vi "SubTemplate2UI.vi"() -> ()   [LabVIEW 2016]
uses:
  Package ResourceControl/ViHandler/ViHandler.ViInfo.ctl
  Message Queue/private/MessageQueue.MessageTypeDef.ctl
  Package ErrorHandling/ErrorHandling.lvclass/ErrorHandling.ctl
  Package ErrorHandling/ErrorHandling.checkForErrorAndHandle.vi
  Package ErrorHandling/ErrorHandling.GetErrorHandler.vi
  <vilib>/Utility/error.llb/Clear Errors.vi
  StringFunctions/StringFunctions_ReplaceAllBlindSigns.vi
  <vilib>/dlg_ctls.llb/Space Constant.vi
  <vilib>/Utility/error.llb/Error Cluster From Error Code.vi
  TimingFunctions/TimingFunctions_getUtcTimestamp.vi
  <vilib>/Utility/error.llb/Trim Whitespace.vi
  <vilib>/Utility/error.llb/Search and Replace Pattern.vi
  Package ErrorHandling/ErrorHandling.addLastErrorToFile.vi
  <vilib>/ErrorRing/Error Ring.xnode
  Package ErrorHandling/ErrorHandling.lvclass
  Package ResourceControl/ViHandler/ViHandler.lvclass
panel:
  out "ViInfoTemp":T1
  # "Batch Conversion"
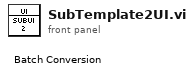
[diagram p1: front panel]
types:
  T1 = typedef "ViHandler.lvclass/ViHandler.ViInfo.ctl" = cluster{"ViName":string, "ViReference":refnum<vi>, "ViQueueName":string}
  T2 = typedef "MessageQueue.MessageTypeDef.ctl" = cluster{"Message":string, "Data":variant}
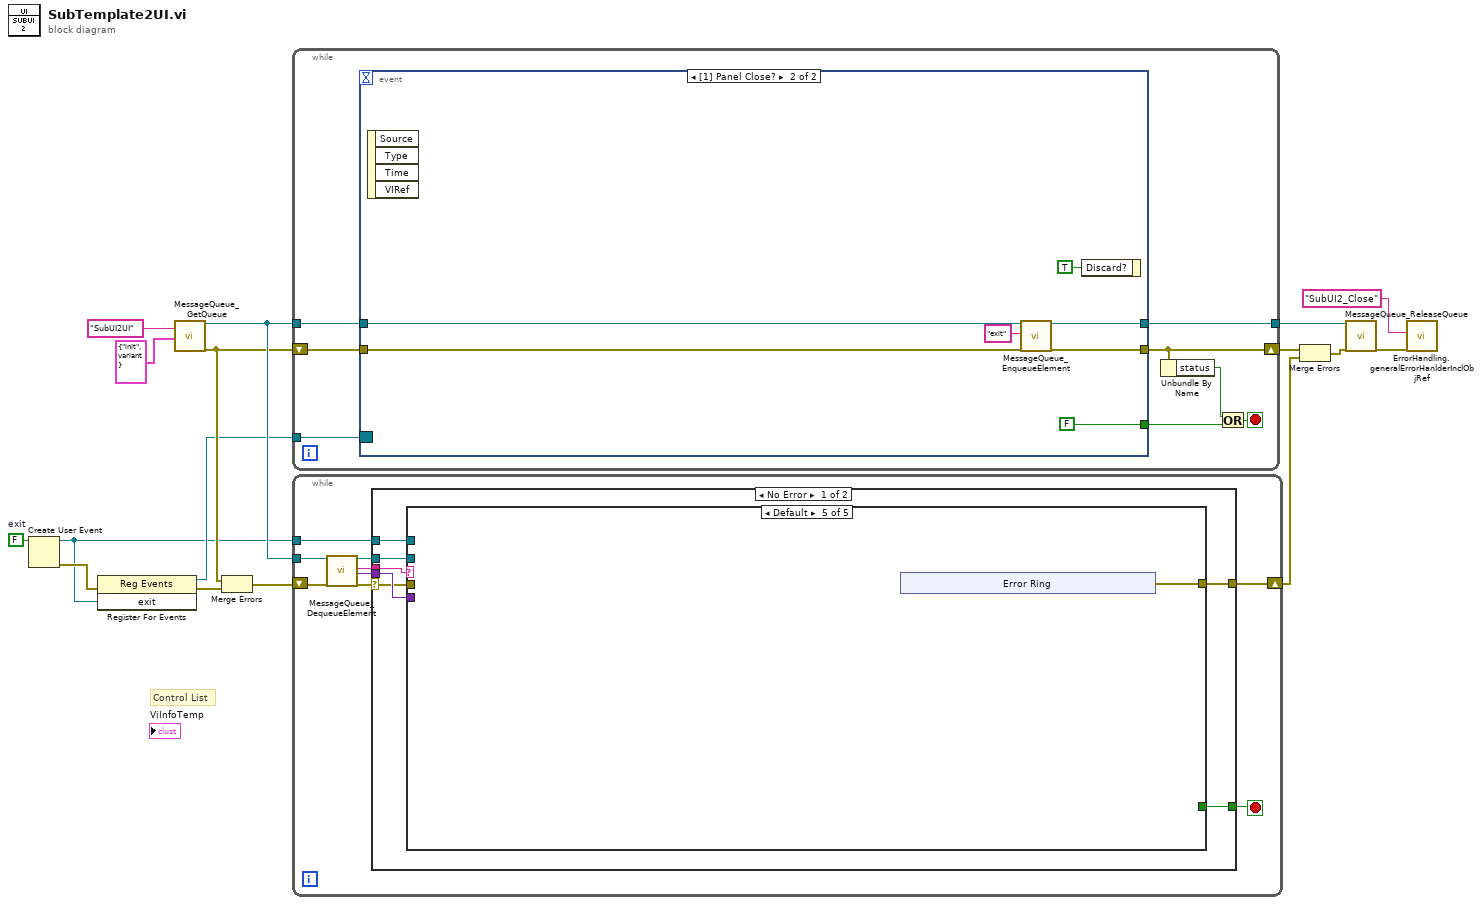
[diagram p0: block diagram]
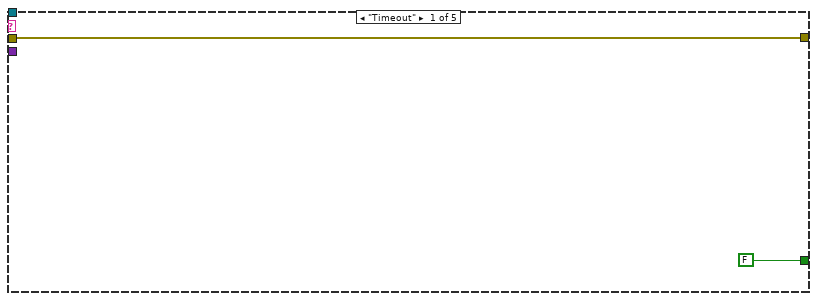
[diagram p2: hidden frame]
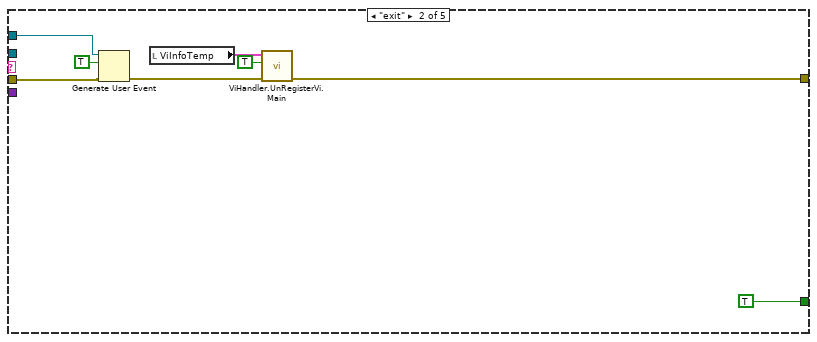
[diagram p3: hidden frame]
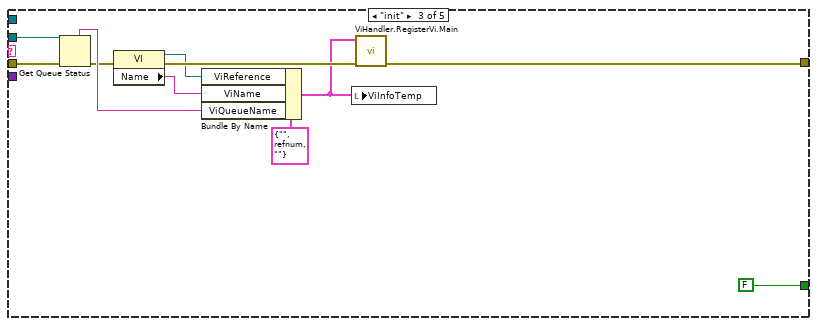
[diagram p4: hidden frame]
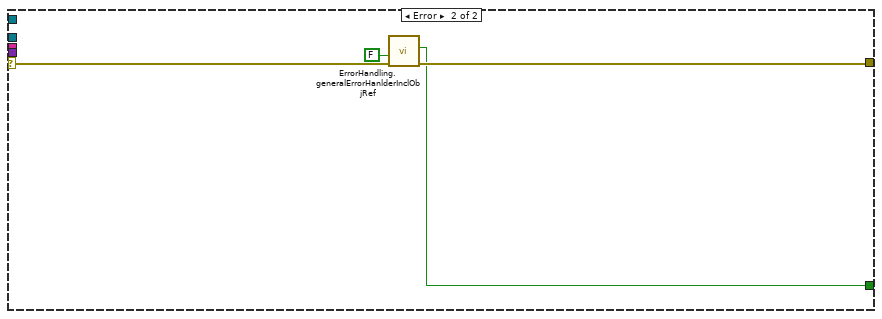
[diagram p6: hidden frame]
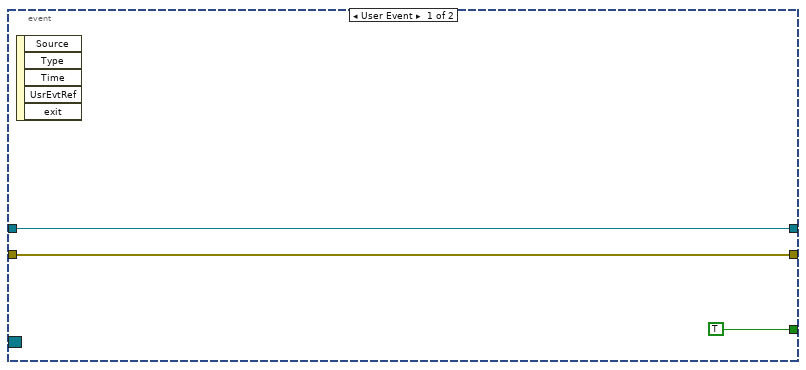
[diagram p7: hidden frame]
diagram:
  w9 = FALSE  # exit
  # "Control List"
  n1 = Create User Event(user event datatype=w9) -> (user event=w7:refnum<user-event>, error out=w8:errorcluster)  [unwired: 1 in]
  n2 = register-events(error in=w8, w7) -> (reference out=w11:refnum<event-registration>, error out=w13:errorcluster)  [unwired: 1 in]
  n3 = call "MessageQueue_GetQueue.vi"("Name"="SubUI2UI", "OptionalInitValue"=T2 {"Message"="init", "Data"=variant}) -> ("QueueOut"=w15:refnum<queue>, "ErrorOut"=w12:errorcluster)  [unwired: 15 in, 1 out]
  n4 = Merge Errors(w12, w13) -> (w10:errorcluster)
  n5 = while {
    tunnel: w15 -> [w24]
    tunnel: [w23] -> w16
    shift-right: [w20] -> w4
    shift-left: w12 -> [w22]
    tunnel: w11 -> [w17]
    stop <- w19 stop-if-true
    n6 = event shown="[1] Panel Close?" {
      selector: w17 -> [_ _]
      dyn-events: _ -> [_ _]
      timeout: _ -> [_ _]
      tunnel: w24 -> [w26 w34]
      tunnel: [w26 w33] -> w23
      tunnel: [w25 w32] -> w20
      tunnel: w22 -> [w25 w31]
      tunnel: [TRUE FALSE] -> w21
      event User Event {
        n7 = event-data() -> ()  [unwired: 1 in, 5 out]
      }
      event Panel Close? {
        n8 = event-data() -> ()  [unwired: 1 in, 4 out]
        n9 = call "MessageQueue_EnqueueElement.vi"("QueueIn"=w34, "Message"="exit", "ErrorIn"=w31) -> ("QueueOut"=w33:refnum<queue>, "ErrorOut"=w32:errorcluster)  [unwired: 15 in]
        n10 = event-data("Discard?"=TRUE) -> ()  [unwired: 1 in, 1 out]
      }
    }
    n11 = Unbundle By Name(w20) -> ("status"=w18:bool)
    n12 = Or(x=w18, y=w21) -> (x .or. y?=w19:bool)
  }
  n13 = while {
    tunnel: w15 -> [w43]
    tunnel: w7 -> [w36]
    shift-right: [w35] -> w5
    shift-left: w10 -> [w37]
    stop <- w38 stop-if-true
    n14 = call "MessageQueue_DequeueElement.vi"("QueueIn"=w43, "ErrorIn"=w37) -> ("QueueOut"=w41:refnum<queue>, "Message"=w40:string, "Data"=w39:variant, "ErrorOut"=w42:errorcluster)  [unwired: 13 in, 1 out]
    n15 = case shown="No Error" w42 {
      selector: w42 -> [w46 w82]
      tunnel: w41 -> [w50 _]
      tunnel: w40 -> [w49 _]
      tunnel: w39 -> [w48 _]
      tunnel: [w47 w80] -> w38
      tunnel: w36 -> [w45 _]
      tunnel: [w44 w81] -> w35
      frame No Error {
        n16 = case shown="Default" w49 {
          tunnel: w50 -> [_ _ w63 _ _]
          tunnel: w48 -> [_ _ _ _ _]
          tunnel: [FALSE TRUE FALSE _ _] -> w47
          tunnel: w46 -> [w51 w58 w64 w72 _]
          tunnel: w45 -> [_ w57 _ _ _]
          tunnel: [w51 w54 w61 w72 w73] -> w44
          frame "Timeout" {
          }
          frame "exit" {
            n17 = Generate User Event(user event=w57, event data cluster=TRUE ("event data"), error in=w58) -> (error out=w55:errorcluster)  [unwired: 1 in, 1 out]
            n18 = local read "ViInfoTemp"() -> (w56:T1)
            n19 = call "ViHandler.UnRegisterVi.Main.vi"("ErrorIn"=w55, "FinalExit?"=TRUE, "ViInfo"=w56) -> ("ErrorOut"=w54:errorcluster)  [unwired: 7 in, 1 out]
          }
          frame "init" {
            n20 = Get Queue Status(queue=w63, error in (no error)=w64) -> (queue name=w69:string, error out=w68:errorcluster)  [unwired: 1 in, 6 out]
            n21 = property class="VI"(error in=w68) -> (reference out=w66:refnum<vi>, error out=w67:errorcluster, "Name"=w65:string)  [unwired: 1 in]
            n22 = Bundle By Name(cluster=T1 {"ViName"="", "ViReference"=refnum, "ViQueueName"=""} ("ViInfo"), "ViReference"=w66, "ViName"=w65, "ViQueueName"=w69) -> (w62:T1)
            n23 = local write "ViInfoTemp"(w62) -> ()
            n24 = call "ViHandler.RegisterVi.Main.vi"("ErrorIn"=w67, "ViInfo"=w62) -> ("ErrorOut"=w61:errorcluster)  [unwired: 9 in]
          }
          frame "UpdateGUI" {
          }
          frame Default {
            n25 = xnode "Error Ring"() -> ("error out"=w73:errorcluster)
          }
        }
      }
      frame Error {
        n26 = call "ErrorHandling.generalErrorHanlderInclObjRef.vi"("error in"=w82, "StopOnError"=FALSE) -> ("error out"=w81:errorcluster, "Stop"=w80:bool)  [unwired: 7 in, 1 out]
      }
    }
  }
  n27 = Merge Errors(w4, w5) -> (w3:errorcluster)
  n28 = call "MessageQueue_ReleaseQueue.vi"("QueueIn"=w16, "ErrorIn"=w3) -> ("ErrorOut"=w2:errorcluster)  [unwired: 15 in, 2 out]
  n29 = call "ErrorHandling.generalErrorHanlderInclObjRef.vi"("error in"=w2, "Comment(optional)"="SubUI2_Close") -> ()  [unwired: 7 in, 3 out]
